vi "Serrure_V2.vi"() -> ()   [LabVIEW 2018]
uses:
  Global 1.vi
panel:
  out "Maximum":dbl
  out "Nb Tentative":dbl
  in  "Ouvrir Button":bool
  out "Rouge":bool
  out "Vert":bool
  out "Compeur":i16
  in  "Boolean 2":bool
  in  "Dial 3":i8(knob) min=0 max=9 scale=0.0..9.0
  in  "Dial 2":i8(knob) min=0 max=9 scale=0.0..9.0
  in  "Dial":i8(knob) min=0 max=9 scale=0.0..9.0
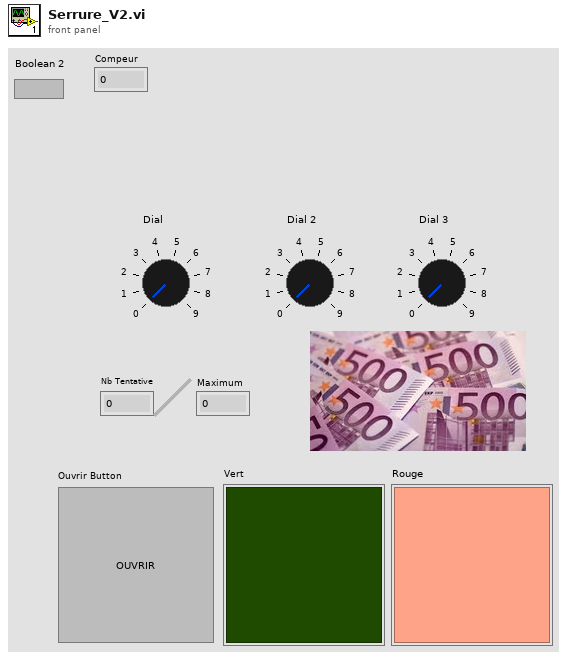
[diagram p1: front panel]
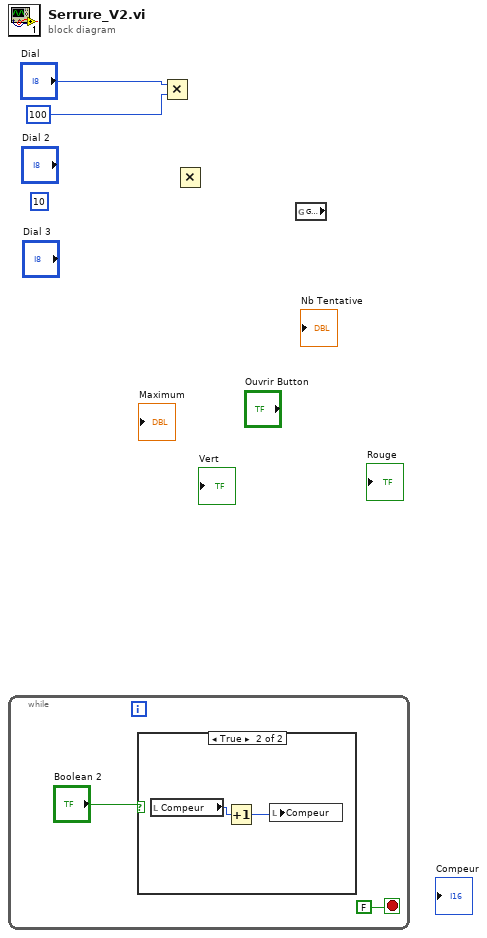
[diagram p0: block diagram]
diagram:
  (unwired) i8 10 ("Dial 2")
  n1 = while {
    stop <- FALSE stop-if-true
    n2 = case shown="True" "Boolean 2" {
      frame False {
      }
      frame True {
        n3 = local read "Compeur"() -> (w5:i16)
        n4 = Increment(x=w5) -> (x+1=w6:i16)
        n5 = local write "Compeur"(w6) -> ()
      }
    }
  }
  n6 = Multiply(x="Dial", y=i8 100 ("Dial")) -> ()  [unwired: 1 out]
  n7 = Multiply() -> ()  [unwired: 2 in, 1 out]
  n8 = global read "Global 1.vi" item#-1() -> ()  [unwired: 1 out]
